vi "Actor Core.vi"(8 "error in":errorcluster, 11 "TCP_serverGUI in":refnum<class "TCP_serverGUI.lvclass">) -> (0 "error out":errorcluster, 3 "Actor out":refnum<class "Actor.lvclass">)   [LabVIEW 2023, in "TCP_serverGUI.lvlib" / "TCP_serverGUI.lvclass"]
doc: "(<B>Filename</B>: Actor Framework.lvlib:Actor.lvclass:Actor Core.vi)\n\nReceives messages to the actor, reacts to them, and initiates any error handling that may shut the actor down.\n\nDescendant classes may override this VI to append parallel tasks for the actor to complete while it handles messages. Overrides use the Call Parent Class Method node."
uses:
  TCP_serverGUI.lvclass
  C:/Program Files (x86)/National Instruments/LabVIEW 2023/vi.lib/ActorFramework/Actor/Actor.lvclass
  <vilib>/ActorFramework/Actor/Actor.lvclass
  TypeDefinitions/ControlReferences.ctl
  TCP_serverGUI.lvclass/TCP_serverGUI.ctl
  <vilib>/ActorFramework/Actor/Actor.lvclass/Actor.ctl
  <vilib>/ActorFramework/Message Enqueuer/Message Enqueuer.lvclass/Message Enqueuer.ctl
  <vilib>/ActorFramework/Message Enqueuer/Init from Existing Queue.vi
  <vilib>/ActorFramework/Message Enqueuer/Enqueue.vi
  TCP_serverGUI Messages/Dissconnect Msg/Dissconnect Msg.lvclass
  C:/Program Files (x86)/National Instruments/LabVIEW 2023/vi.lib/ActorFramework/Message/Message.lvclass
  TCP_ServerWithGUI Messages/ShutDown Msg/ShutDown Msg.lvclass
  <vilib>/ActorFramework/Message Priority Queue/Priority Enqueue.vi
  <vilib>/ActorFramework/Message Enqueuer/Message Enqueuer.lvclass
panel:
  in  "Stop Server Button":bool
  in  "Dissconnect Button":bool
  out "Number of connections":i32
  in  "Connections":i32[](listbox)
  out "Number of errors":u32
  out "file number":u32
  out "Error log file":path
  out "Server":string
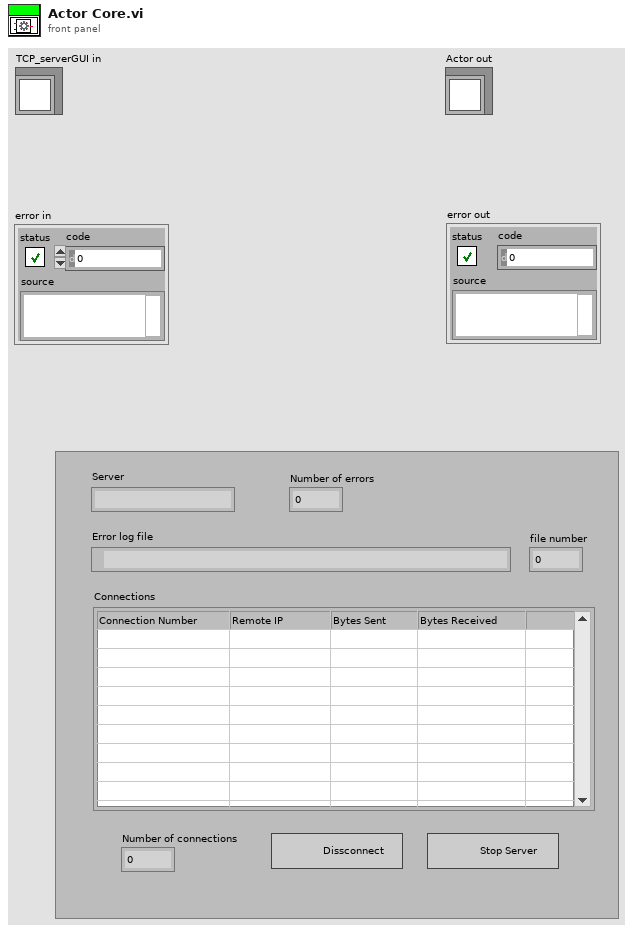
[diagram p1: front panel]
types:
  T1 = typedef "TCP_serverGUI.lvlib/TCP_serverGUI.lvclass/ControlReferences.ctl" = cluster{"Server ":refnum<vi>, "Number of errors":refnum<vi>, "Error log file":refnum<vi>, "file number":refnum<vi>, "Connections":refnum<vi>, "Number of connections":refnum<vi>}
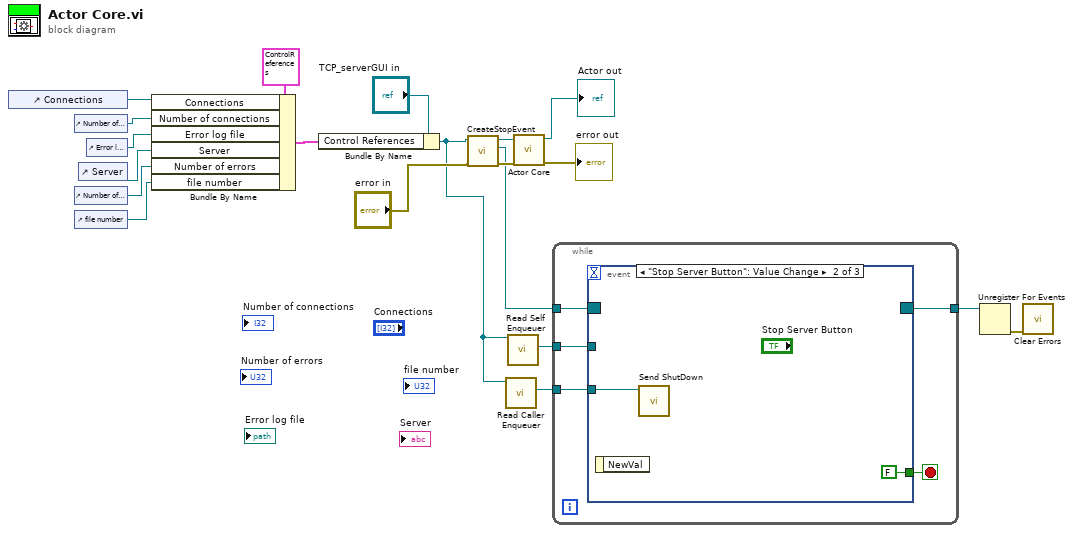
[diagram p0: block diagram]
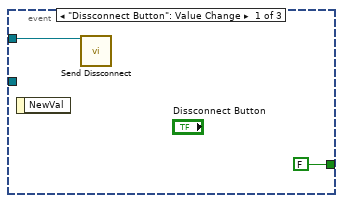
[diagram p2: hidden frame]
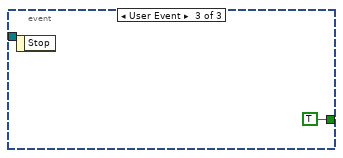
[diagram p3: hidden frame]
diagram:
  n1 = control-ref of="Connections"() -> (w4:refnum<vi>)
  n2 = control-ref of="Number of connections"() -> (w3:refnum<vi>)
  n3 = control-ref of="Number of errors"() -> (w9:refnum<vi>)
  n4 = control-ref of="file number"() -> (w6:refnum<vi>)
  n5 = control-ref of="Server"() -> (w10:refnum<vi>)
  n6 = control-ref of="Error log file"() -> (w11:refnum<vi>)
  n7 = Bundle By Name(cluster=T1 {"Server "=refnum, "Number of errors"=refnum, "Error log file"=refnum, "file number"=refnum, "Connections"=refnum, "Number of connections"=refnum} ("Control References"), "Connections"=w4, "Number of connections"=w3, "Error log file"=w11, "Server"=w10, "Number of errors"=w9, "file number"=w6) -> (w7:T1)
  n8 = Bundle By Name(cluster="TCP_serverGUI in", "Control References"=w7) -> (w2:refnum<class "TCP_serverGUI.lvclass">)
  n9 = call "CreateStopEvent.vi"("error in (no error)"="error in", "TCP_serverGUI in"=w2) -> ("error out"=w17:errorcluster, "Event Registration Refnum"=w15:refnum<event-registration>, "TCP_serverGUI out"=w18:refnum<class "TCP_serverGUI.lvclass">)  [unwired: 7 in]
  n10 = call <vilib>:"Read Caller Enqueuer.vi"("Actor"=w2) -> ("Caller Enqueuer"=w5:refnum<class "Message Enqueuer.lvclass">)  [unwired: 10 in]
  n11 = call <vilib>:"Read Self Enqueuer.vi"("Actor"=w2) -> ("Self Enqueuer"=w1:refnum<class "Message Enqueuer.lvclass">)  [unwired: 10 in]
  n12 = call-parent "Actor Core.vi"("error in"=w17, "Actor in"=w18) -> ("error out"=→"error out":errorcluster, "Actor out"=→"Actor out":refnum<class "Actor.lvclass">)  [unwired: 8 in]
  n13 = while {
    tunnel: w15 -> [w24]
    tunnel: [w23] -> w14
    tunnel: w5 -> [w22]
    tunnel: w1 -> [w21]
    stop <- w25 stop-if-true
    n14 = event shown="[1] \"Stop Server Button\": Value Change" {
      selector: w24 -> [_ _ _]
      dyn-events: [_ _ _] -> w23
      timeout: _ -> [_ _ _]
      tunnel: [FALSE FALSE TRUE] -> w25
      tunnel: w22 -> [_ w28 _]
      tunnel: w21 -> [w26 _ _]
      event "Dissconnect Button": Value Change {
        n15 = event-data() -> ()  [unwired: 1 in, 1 out]
        n16 = call "Send Dissconnect.vi"("Message Enqueuer"=w26) -> ()  [unwired: 9 in, 2 out]
      }
      event "Stop Server Button": Value Change {
        n17 = event-data() -> ()  [unwired: 1 in, 1 out]
        n18 = call "Send ShutDown.vi"("Message Enqueuer"=w28) -> ()  [unwired: 9 in, 2 out]
      }
      event User Event {
        n19 = event-data() -> ()  [unwired: 1 in, 1 out]
      }
    }
  }
  n20 = Unregister For Events(event registration refnum=w14) -> (error out=w13:errorcluster)  [unwired: 1 in]
  n21 = call <vilib>:"Clear Errors.vi"("error in (no error)"=w13) -> ()  [unwired: 5 in, 2 out]
